vi "FitsWriteSGL.vi"(6 "Array":sgl[](array[numeric])=[0.0071213036, 0.0058665383, 0.006181328, 0.009479352, 0.0040471675, 0.003067414, 0.004592165, 0.00427941, 0.0027120172, 0.004816928, 0.009925612, 0.008061036, 0.0017669186, 0.0010894345, 0.0021162627, 0.0048869033, 0.006004254, 0.0060450956, 0.0025992065, -0.0008630056, 0.0053265993, 0.015476205, 0.01445547, 0.007017845, 0.0011118925, -0.0024843821, -0.0008969588, 0.0014443859, 0.0043489733, 0.0063615725, 0.007806599, 0.0045245844, 0.0008055465, -0.002944382, -0.0058082803, 0.005272431, 0.020363992, 0.020071195, 0.011525899, 0.00599592, -0.1038012, -0.105127014, -0.099082254, -0.07519699, -0.019978138, 0.030296674, 0.088178515, 0.116585694, 0.12907822, 0.10991168, 0.06561601, -0.020711435, -0.20185162, -0.61261475, -0.3005922, 0.9175789, 0.4203767, 0.143611, 0.01524742, -0.057749126] format="%.2f", 7 "ref":u64, 8 "error in (no error)":errorcluster, 9 "nelem":i32, 10 "firstel":i32, 11 "CFitsIO in":refnum<class "CFitsIO.lvclass">) -> (0 "error out":errorcluster, 3 "CFitsIO out":refnum<class "CFitsIO.lvclass">)   [LabVIEW 2016, in "CFitsIO.lvclass"]
uses:
  CFitsIO.lvclass
panel:
  out "result":i32
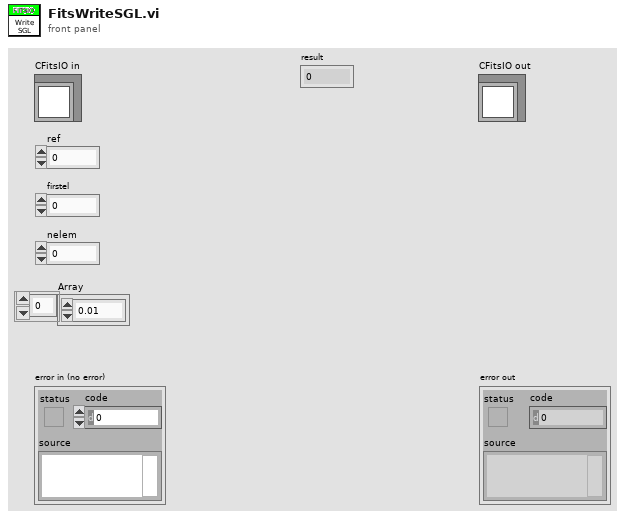
[diagram p1: front panel]
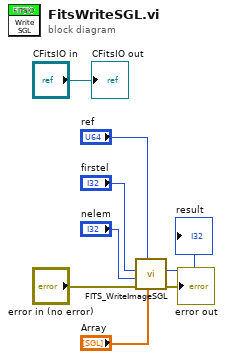
[diagram p0: block diagram]
diagram:
  n1 = call "FITS_WriteImageSGL.vi"("Array"="Array", "ref"="ref", "error in"="error in (no error)", "nelem"="nelem", "firstel"="firstel") -> ("error out"=→"error out":errorcluster, "result"=→"result":i32)  [unwired: 5 in]
  "CFitsIO out" <- "CFitsIO in"
